vi "Async Action.vi"(8 "error in (no error)":errorcluster, 9 "Message Data":variant, 10 "Message":string, 11 "Asynchronous Action In":refnum<class "Customer.lvclass">) -> (0 "error out":errorcluster, 3 "Asynchronous Action Out":refnum<class "Customer.lvclass">)   [LabVIEW 2020, in "Customer.lvclass"]
doc: "The specific action implemented in the asynchronous action. Multiple different actions may be supported by using the Message and Message Data input to separate them. Any number of actions may run in parallell running the same or different actions. If this method throws an error, the error will be sent to the error handler configured for the process. \nCare needs to be taken so that this action is cancelled if the process is stopped. This may be detected by e.g. observing the Lifecycle: Stopped/Finished broadcast or polling the Get Lifecycle State.vi."
uses:
  Customer.lvclass
  C:/Program Files (x86)/National Instruments/LabVIEW 2020/vi.lib/Asteme/Triarc Framework/Process/Process.lvclass
  Customer.lvclass/Customer.ctl
  <vilib>/Asteme/Triarc Framework/Application/Application.lvclass
  <vilib>/Asteme/Triarc Framework/Process/Process.lvclass/Process.ctl
  <vilib>/Asteme/Triarc Framework/Application/Application.lvclass/Application.ctl
  <vilib>/Asteme/Triarc Framework/Process/Public/Lifecycle/Get Lifecycle State.vi
  <vilib>/Asteme/Triarc Framework/Process/Protected/Messaging/Enqueue Message.vi
  <vilib>/Asteme/Triarc Framework/Process/Private/SubVIs/Wait for finish.vi
  <vilib>/Asteme/Triarc Framework/Process/Private/SubVIs/Set Lifecycle State.vi
  <vilib>/Utility/error.llb/Clear Errors.vi
  <vilib>/AdvancedString/1D String Array to Delimited String.vi
  <vilib>/Utility/error.llb/Error Cluster From Error Code.vi
  <vilib>/Asteme/Triarc Framework/Process/Process.lvclass
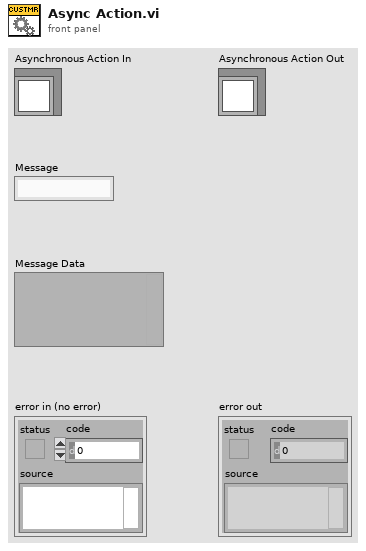
[diagram p1: front panel]
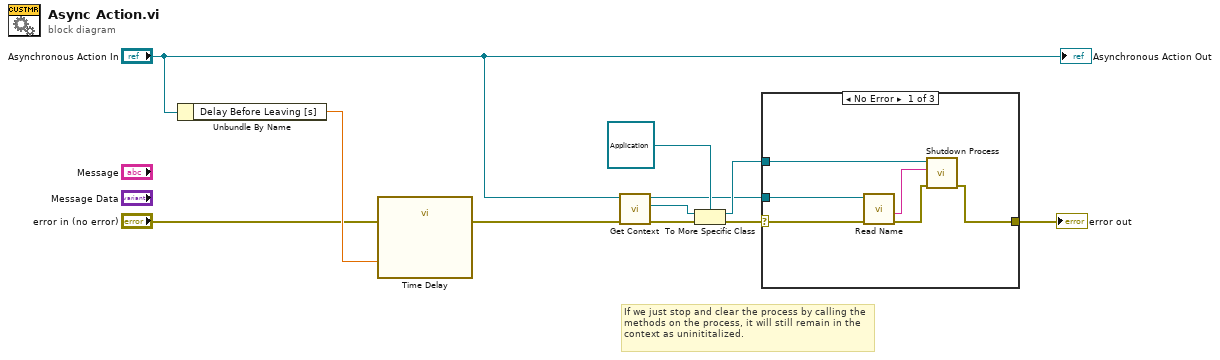
[diagram p0: block diagram]
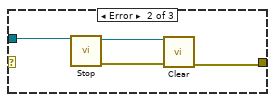
[diagram p2: hidden frame]
diagram:
  # "If we just stop and clear the process by calling the methods on the process, it will still remain in the context as uninititalized."
  n1 = Unbundle By Name("Asynchronous Action In") -> ("Delay Before Leaving [s]"=w3:dbl)
  n2 = call "Time Delay"("error in (no error)"="error in (no error)", "Delay Time (s)"=w3) -> ("error out"=w1:errorcluster)  [unwired: 9 in]
  n3 = call <vilib>:"Get Context.vi"("error in (no error)"=w1, "Process In"="Asynchronous Action In") -> ("error out"=w11:errorcluster, "Context"=w10:refnum<class "Process.lvclass">, "Process Out"=w6:refnum<class "Customer.lvclass">)  [unwired: 6 in, 1 out]
  n4 = To More Specific Class(target class=refnum<class "Application.lvclass"> refnum ("TF.lvlib:Application.lvclass"), reference=w10, error in=w11) -> (specific class reference=w7:refnum<class "Application.lvclass">, error out=w8:errorcluster)
  n5 = case shown="No Error" w8 {
    selector: w8 -> [w17 _ w22]
    tunnel: w7 -> [w16 _ _]
    tunnel: w6 -> [w15 w19 _]
    tunnel: [w12 w18 w22] -> w5
    frame No Error {
      n6 = call-dynamic "Read Name.vi"("error in (no error)"=w17, "Process In"=w15) -> ("error out"=w13:errorcluster, "Name"=w14:string)  [unwired: 6 in, 2 out]
      n7 = call <vilib>:"Shutdown Process.vi"("error in (no error)"=w13, "Process Name"=w14, "Rig In"=w16) -> ("error out"=w12:errorcluster)  [unwired: 7 in, 1 out]
    }
    frame Error {
      n8 = call <vilib>:"Stop.vi"("Process In"=w19) -> ("error out"=w20:errorcluster, "Process Out"=w21:refnum<class "Customer.lvclass">)  [unwired: 8 in, 1 out]
      n9 = call-dynamic "Clear.vi"("error in (no error)"=w20, "View In"=w21) -> ("error out"=w18:errorcluster)  [unwired: 9 in]
    }
    frame Default {
    }
  }
  "error out" <- w5
  "Asynchronous Action Out" <- "Asynchronous Action In"
